vi "Laplacian.vi"() -> ()   [LabVIEW 2025]
uses:
  <vilib>/Math Plots/3D Math Plots/3D Contour/3D Contour XCtrl/3D Contour.xctl
  <vilib>/Math Plots/3D Math Plots/3D Contour/3D Contour Datatype/Public/Plot Helper (Matrix).vi
  <vilib>/Math Plots/3D Math Plots/3D Contour/3D Contour Datatype/3D Contour Datatype.lvclass
panel:
  in  "Uinf":dbl
  out "3D Contour":refnum<class "3D Plot Datatype.lvclass">[](xcontrol)
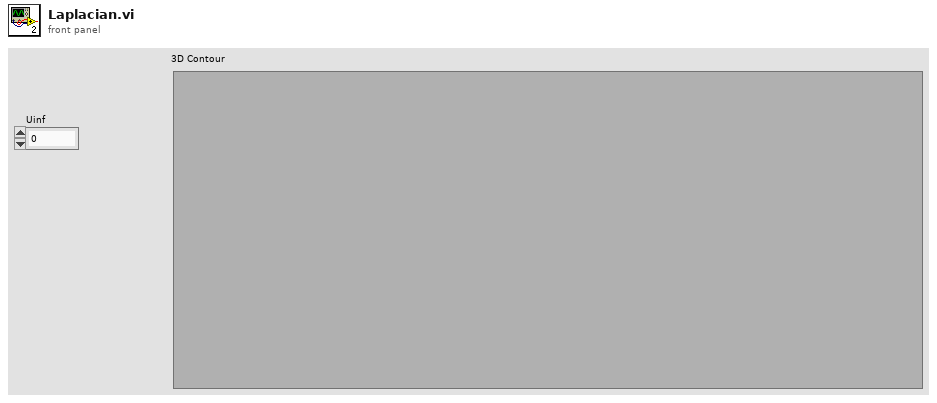
[diagram p1: front panel]
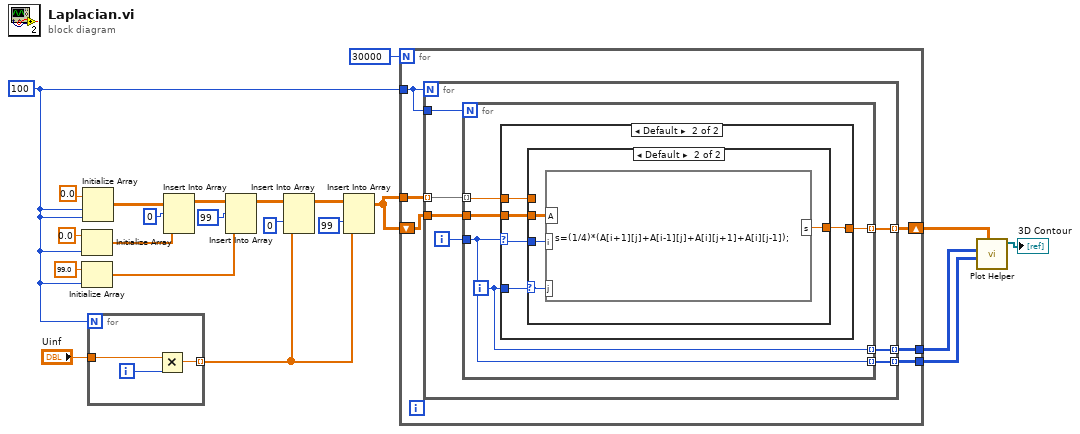
[diagram p0: block diagram]
diagram:
  w1 = 100
  n1 = Initialize Array(0.0, w1) -> (w15:dbl[])
  n2 = Initialize Array(99.0, w1) -> (w11:dbl[])
  n3 = Initialize Array(0.0, w1, w1) -> (w18:dbl[][])
  n4 = for {
    N: w1 -> [_]
    tunnel: "Uinf" -> [w24]
    tunnel: [w23] -> w5 mode=indexing
    i -> [w25]
    n5 = Multiply(x=w24, y=w25) -> (x*y=w23:dbl)
  }
  n6 = Insert Into Array(array=w18, index (row)=0, new element=w15) -> (w12:dbl[][])  [unwired: 1 in]
  n7 = Insert Into Array(array=w12, index (row)=99, new element=w11) -> (w9:dbl[][])  [unwired: 1 in]
  n8 = Insert Into Array(array=w9, index (col)=0 ("index (row)"), new element=w5) -> (w6:dbl[][])  [unwired: 1 in]
  n9 = Insert Into Array(array=w6, index (col)=99 ("index (row)"), new element=w5) -> (w4:dbl[][])  [unwired: 1 in]
  n10 = for {
    N: 30000 -> [_]
    tunnel: w4 -> [w31]
    shift-right: [w28] -> w21
    shift-left: w4 -> [w30]
    tunnel: w1 -> [w29]
    tunnel: [w27] -> w3
    tunnel: [w26] -> w2
    n11 = for {
      N: w29 -> [_]
      tunnel: w31 -> [w38] mode=indexing
      tunnel: [w36] -> w28 mode=indexing
      tunnel: w30 -> [w35]
      tunnel: w29 -> [w34]
      tunnel: [w33] -> w27 mode=indexing
      tunnel: [w32] -> w26 mode=indexing
      i -> [w37]
      n12 = for {
        N: w34 -> [_]
        tunnel: w38 -> [w42] mode=indexing
        tunnel: w37 -> [w39]
        tunnel: [w43] -> w36 mode=indexing
        tunnel: w35 -> [w41]
        tunnel: [w40] -> w33 mode=indexing
        tunnel: [w39] -> w32 mode=indexing
        i -> [w40]
        n13 = case shown="Default" w39 {
          selector: w39 -> [_ w49]
          tunnel: [w44 w47] -> w43
          tunnel: w42 -> [w44 w45]
          tunnel: w40 -> [_ w46]
          tunnel: w41 -> [_ w48]
          frame 0, 99 {
          }
          frame Default {
            n14 = case shown="Default" w46 {
              selector: w46 -> [_ w51]
              tunnel: w49 -> [_ w54]
              tunnel: w48 -> [_ w53]
              tunnel: [w50 w52] -> w47
              tunnel: w45 -> [w50 _]
              frame 0, 99 {
              }
              frame Default {
                n15 = formula code="s=(1/4)*(A[i+1][j]+A[i-1][j]+A[i][j+1]+A[i][j-1]);"("A"=w53, "i"=w54, "j"=w51) -> ("s"=w52:dbl)
              }
            }
          }
        }
      }
    }
  }
  n16 = call-poly <vilib>:"Plot Helper.vi"("z matrix"=w21, "y matrix"=w2, "x matrix"=w3) -> ("3D Plot lvclass Array out"=→"3D Contour":refnum<class "3D Plot Datatype.lvclass">[])  [unwired: 3 in, 5 out]
